vi "Continuous FM Test.vi"() -> ()   [LabVIEW 2015]
uses:
  <vilib>/sound2/lvsound2.llb/Sampling Mode.ctl
  <vilib>/sound2/lvsound2.llb/Sound Data Format.ctl
  Waveform VIs/FM Sweep VIs/SFM-Params.ctl
  <vilib>/sound2/lvsound2.llb/Sound Output Write (DBL Single).vi
panel:
  in  "Slide":dbl(slide)=20.0 min=1.0 max=20.0 step=1.0 scale=1.0..20.0
  in  "Sampling Rate (Hz)":dbl=20000.0
  out "Time":dbl[](graph)
  in  "Stop":bool
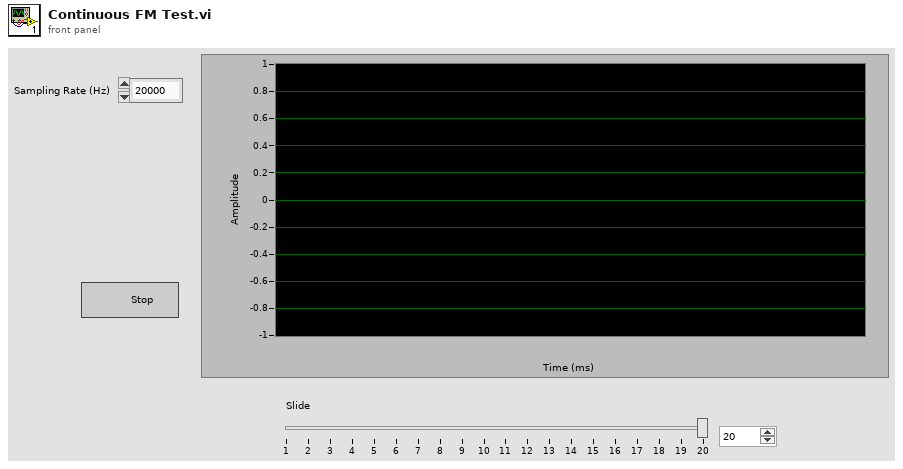
[diagram p1: front panel]
types:
  T1 = typedef "SFM-Params.ctl" = cluster{"ModArg":dbl, "MainArg":dbl, "FMod":dbl, "Fcarrier":dbl, "Fdepth":dbl}
  T2 = typedef "Sound Data Format.ctl" = cluster{"sample rate (S/s)":dbl, "number of channels":i32, "bits per sample":i32}
  T3 = typedef "Sampling Mode.ctl" = i32
  T4 = typedef "Sound Output Task ID.ctl" = u32
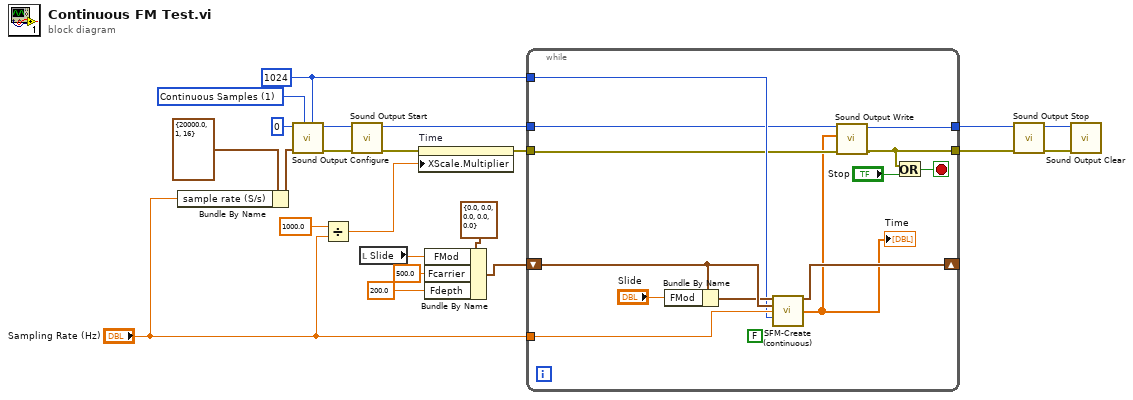
[diagram p0: block diagram]
diagram:
  w7 = 1024 ("number of samples/ch")
  w21 = T3 1 items=["Finite Samples", "Continuous Samples"] ("sample mode")
  n1 = Bundle By Name(cluster=T2 {"sample rate (S/s)"=20000.0, "number of channels"=1, "bits per sample"=16} ("sound format"), "sample rate (S/s)"="Sampling Rate (Hz)") -> (w10:T2)
  n2 = call <vilib>:"Sound Output Configure.vi"("number of samples/ch"=w7, "sample mode"=w21, "sound format"=w10, "device ID"=u32 0) -> ("error out"=w19:errorcluster, "task ID"=w18:T4)  [unwired: 6 in]
  n3 = Divide(x=1000.0, y="Sampling Rate (Hz)") -> (x/y=w8:dbl)
  n4 = call <vilib>:"Sound Output Start.vi"("error in (no error)"=w19, "task ID"=w18) -> ("error out"=w12:errorcluster, "task ID out"=w17:T4)  [unwired: 8 in]
  n5 = local read "Slide"() -> (w6:dbl)
  n6 = property on="Time" class="WFGraph (strict)"(error in=w12, "XScale.Multiplier"=w8) -> (error out=w11:errorcluster)  [unwired: 1 in, 1 out]
  n7 = Bundle By Name(cluster=T1 {"ModArg"=0.0, "MainArg"=0.0, "FMod"=0.0, "Fcarrier"=0.0, "Fdepth"=0.0} ("Out"), "FMod"=w6, "Fcarrier"=500.0, "Fdepth"=200.0) -> (w3:T1)
  n8 = while {
    tunnel: w11 -> [w25]
    tunnel: w17 -> [w28]
    tunnel: [w26] -> w16
    tunnel: [w27] -> w15
    tunnel: w7 -> [w29]
    shift-right: [w31] -> _
    shift-left: w3 -> [w33]
    tunnel: "Sampling Rate (Hz)" -> [w30]
    stop <- w34 stop-if-true
    (unwired) FALSE ("Original method?")
    n9 = Bundle By Name(cluster=w33, "FMod"="Slide") -> (w32:T1)
    n10 = call "SFM-Create (continuous).vi"("New"=w32, "Old"=w33, "Fs (Hz)"=w30, "Npts"=w29) -> ("Out"=w31:T1, "Y"=w24:dbl[])  [unwired: 10 in]
    "Time" <- w24
    n11 = call-poly <vilib>:"Sound Output Write.vi"("error in (no error)"=w25, "data"=w24, "task ID"=w28) -> ("error out"=w26:errorcluster, "task ID out"=w27:T4)  [unwired: 7 in]
    n12 = Or(x=w26, y="Stop") -> (x .or. y?=w34:bool)
  }
  n13 = call <vilib>:"Sound Output Stop.vi"("error in (no error)"=w16, "task ID"=w15) -> ("error out"=w14:errorcluster, "task ID out"=w13:T4)  [unwired: 8 in]
  n14 = call <vilib>:"Sound Output Clear.vi"("error in (no error)"=w14, "task ID"=w13) -> ()  [unwired: 9 in, 1 out]
